vi "Update ROI.vi"(8 "error in (no error)":errorcluster, 11 "Detail Graph in":refnum<class "Detail Graph.lvclass">) -> (0 "error out":errorcluster, 3 "Detail Graph out":refnum<class "Detail Graph.lvclass">)   [LabVIEW 2023, in "Detail Graph.lvclass"]
uses:
  Detail Graph.lvclass
  Base Graph/Base Graph.lvclass/Base Graph.ctl
  Detail Graph.lvclass/Detail Graph.ctl
  Base Graph/Base Graph.lvclass
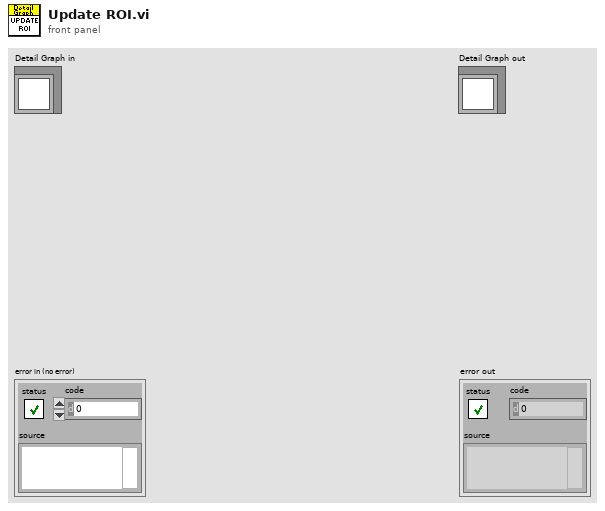
[diagram p1: front panel]
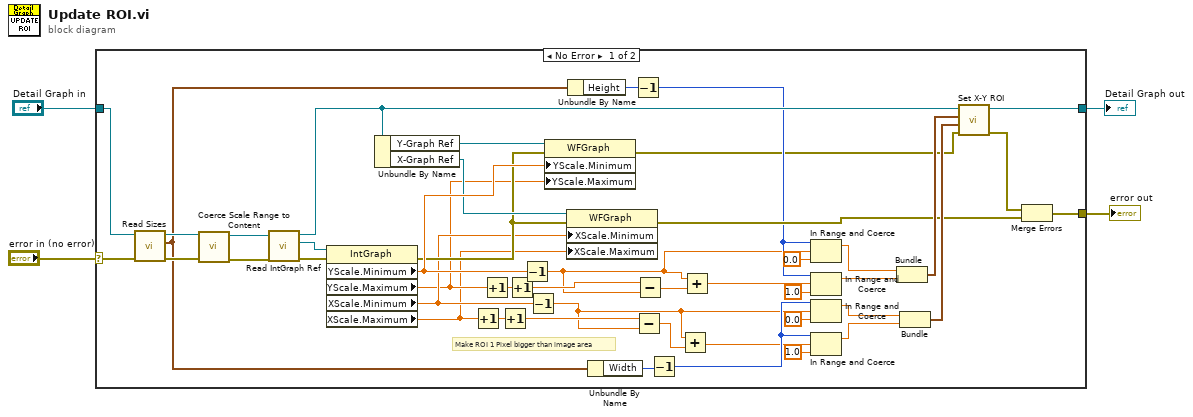
[diagram p0: block diagram]
diagram:
  n1 = case shown="No Error" "error in (no error)" {
    selector: "error in (no error)" -> [w36 w52]
    tunnel: [w38 w52] -> w3
    tunnel: [w48 w51] -> w1
    tunnel: "Detail Graph in" -> [w28 w51]
    frame No Error {
      # "Make ROI 1 Pixel bigger than image area"
      n2 = call "Read Sizes.vi"("error in (no error)"=w36, "TG Base Graph in"=w28) -> ("error out"=w29:errorcluster, "Sizes"=w22:cluster{"Height":u32, "Width":u32}, "TG Base Graph out"=w27:refnum<class "Detail Graph.lvclass">)  [unwired: 7 in]
      n3 = call "Coerce Scale Range to Content.vi"("error in (no error)"=w29, "Base Graph in"=w27) -> ("error out"=w35:errorcluster, "Base Graph out"=w34:refnum<class "Detail Graph.lvclass">)  [unwired: 8 in]
      n4 = call "Read IntGraph Ref.vi"("error in (no error)"=w35, "TG Base Graph in"=w34) -> ("error out"=w49:errorcluster, "IntGraph Ref"=w50:refnum<vi>, "TG Base Graph out"=w44:refnum<class "Detail Graph.lvclass">)  [unwired: 7 in]
      n5 = property on="Property Node" class="IntGraph"(reference=w50, error in=w49) -> (error out=w40:errorcluster, "YScale.Minimum"=w42:dbl, "YScale.Maximum"=w31:dbl, "XScale.Minimum"=w39:dbl, "XScale.Maximum"=w30:dbl)  [unwired: 1 out]
      n6 = Unbundle By Name(w44) -> ("Y-Graph Ref"=w43:refnum<vi>, "X-Graph Ref"=w41:refnum<vi>)
      n7 = Increment(x=w30) -> (x+1=w32:dbl)
      n8 = Increment(x=w31) -> (x+1=w33:dbl)
      n9 = Increment(x=w32) -> (x+1=w26:dbl)
      n10 = Increment(x=w33) -> (x+1=w25:dbl)
      n11 = Decrement(x=w42) -> (x-1=w6:dbl)
      n12 = Decrement(x=w39) -> (x-1=w9:dbl)
      n13 = property on="Property Node" class="WFGraph"(reference=w43, error in=w40, "YScale.Minimum"=w42, "YScale.Maximum"=w31) -> (error out=w5:errorcluster)  [unwired: 1 out]
      n14 = property on="Property Node" class="WFGraph"(reference=w41, error in=w40, "XScale.Minimum"=w39, "XScale.Maximum"=w30) -> (error out=w37:errorcluster)  [unwired: 1 out]
      n15 = Unbundle By Name(w22) -> ("Height"=w23:u32)
      n16 = Unbundle By Name(w22) -> ("Width"=w21:u32)
      n17 = Decrement(x=w23) -> (x-1=w12:u32)
      n18 = Subtract(x=w26, y=w9) -> (x-y=w11:dbl)
      n19 = Subtract(x=w25, y=w6) -> (x-y=w7:dbl)
      n20 = Decrement(x=w21) -> (x-1=w17:u32)
      n21 = Add(x=w9, y=w11) -> (x+y=w10:dbl)
      n22 = Add(x=w6, y=w7) -> (x+y=w8:dbl)
      n23 = In Range and Coerce(upper limit=w12, x=w6, lower limit=0.0) -> (coerced(x)=w24:dbl)  [unwired: 1 out]
      n24 = In Range and Coerce(upper limit=w12, x=w8, lower limit=1.0) -> (coerced(x)=w15:dbl)  [unwired: 1 out]
      n25 = In Range and Coerce(upper limit=w17, x=w9, lower limit=0.0) -> (coerced(x)=w20:dbl)  [unwired: 1 out]
      n26 = In Range and Coerce(upper limit=w17, x=w10, lower limit=1.0) -> (coerced(x)=w14:dbl)  [unwired: 1 out]
      n27 = Bundle("lower limit"=w24, "lower limit"=w15) -> (w46:cluster{"lower limit":dbl, "lower limit":dbl})  [unwired: 1 in]
      n28 = Bundle("lower limit"=w20, "lower limit"=w14) -> (w47:cluster{"lower limit":dbl, "lower limit":dbl})  [unwired: 1 in]
      n29 = call-dynamic "Set X-Y ROI.vi"("error in (no error)"=w5, "ROI X"=w47, "ROI Y"=w46, "TG Base Graph in"=w44) -> ("error out"=w45:errorcluster, "TG Base Graph out"=w48:refnum<class "Detail Graph.lvclass">)  [unwired: 6 in]
      n30 = Merge Errors(w45, w37) -> (w38:errorcluster)
    }
    frame Error {
    }
  }
  "error out" <- w3
  "Detail Graph out" <- w1
